vi "Format Setup String.vi"(0 "TCS in":refnum<class "TCS.lvclass">, 1 "On&G 0":T1, 2 "On&G 1":T1, 3 "On&G 2":T1, 4 "On&G 3":T1, 5 "error in (no error)":errorcluster) -> (14 "TCS out":refnum<class "TCS.lvclass">, 17 "Setup string":string, 19 "error out":errorcluster)   [LabVIEW 2016, in "TCS.lvclass"]
uses:
  Lib.llb/TCS.lvclass
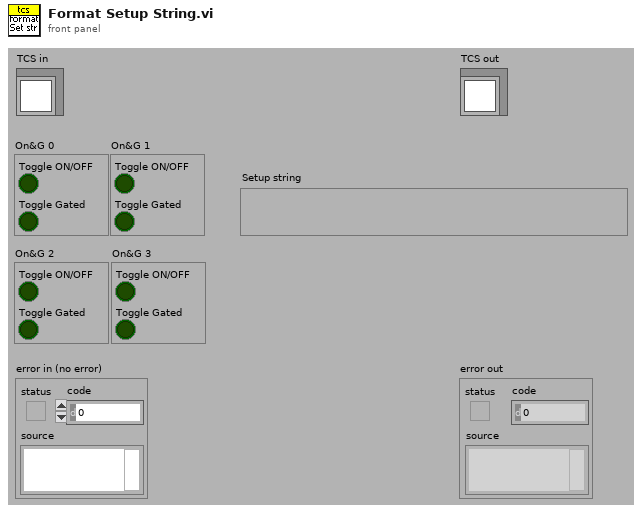
[diagram p1: front panel]
types:
  T1 = cluster{"Toggle ON/OFF":bool, "Toggle Gated":bool}
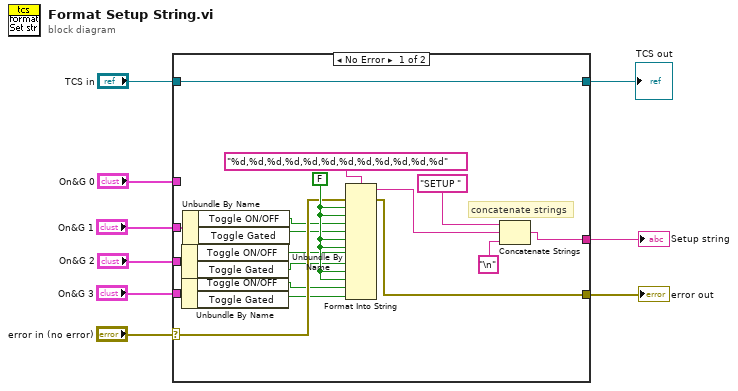
[diagram p0: block diagram]
diagram:
  n1 = case shown="No Error" "error in (no error)" {
    selector: "error in (no error)" -> [w20 w29]
    tunnel: "TCS in" -> [w27 w28]
    tunnel: "On&G 0" -> [_ _]
    tunnel: "On&G 1" -> [w18 _]
    tunnel: "On&G 2" -> [w17 _]
    tunnel: "On&G 3" -> [w16 _]
    tunnel: [w27 w28] -> w4
    tunnel: [w24 _] -> w3
    tunnel: [w19 w29] -> w2
    frame No Error {
      w22 = FALSE
      # "concatenate strings"
      n2 = Unbundle By Name(w17) -> ("Toggle ON/OFF"=w13:bool, "Toggle Gated"=w12:bool)
      n3 = Unbundle By Name(w16) -> ("Toggle ON/OFF"=w11:bool, "Toggle Gated"=w10:bool)
      n4 = Unbundle By Name(w18) -> ("Toggle ON/OFF"=w15:bool, "Toggle Gated"=w14:bool)
      n5 = Format Into String(format string="%d,%d,%d,%d,%d,%d,%d,%d,%d,%d,%d,%d", error in=w20, w22, w22, w15, w14, w22, w22, w13, w12, w22, w22, w11, w10) -> (resulting string=w21:string, error out=w19:errorcluster)  [unwired: 1 in]
      n6 = Concatenate Strings("SETUP ", w21, "\n") -> (w24:string)
    }
    frame Error {
    }
  }
  "error out" <- w2
  "TCS out" <- w4
  "Setup string" <- w3
